vi "Ultramat 23 AFCO Calculations Sub.vi"(7 "CO2 Air Free-Ultimate (%)":dbl, 8 "error in (no error)":errorcluster, 10 "CO2 (%)":dbl, 11 "CO (PPMv)":dbl) -> (0 "error out":errorcluster, 3 "AFCO Data":string[][](array[string]))   [LabVIEW 2023]
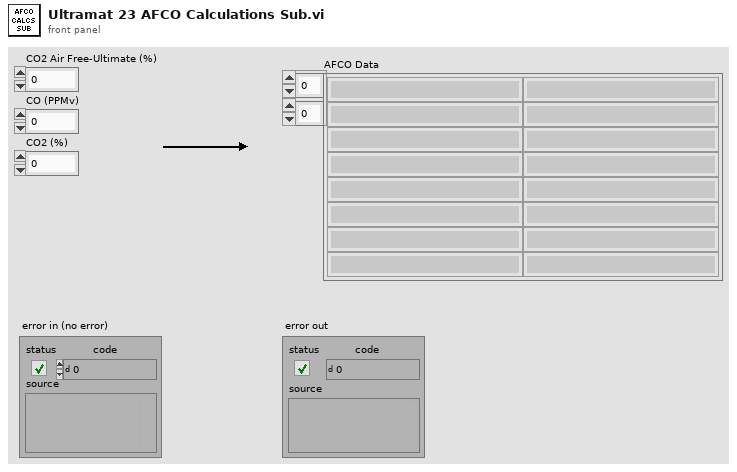
[diagram p1: front panel]
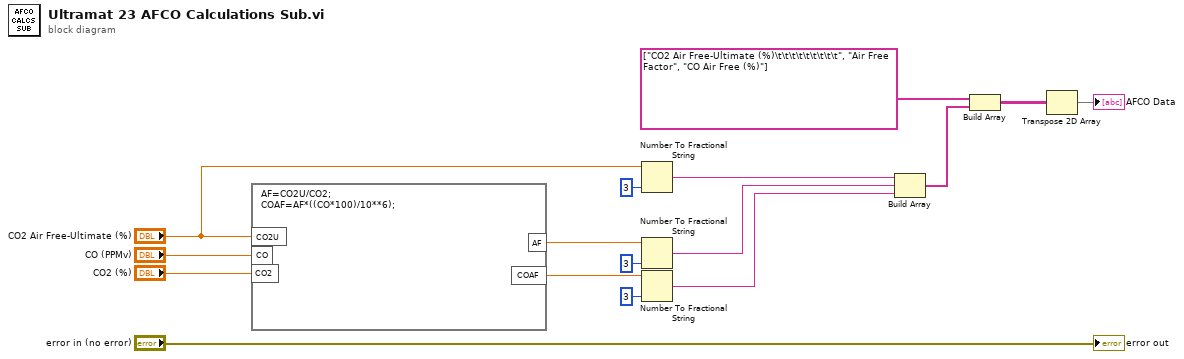
[diagram p0: block diagram]
diagram:
  n1 = formula code="AF=CO2U/CO2;\nCOAF=AF*((CO*100)/10**6);"("CO2U"="CO2 Air Free-Ultimate (%)", "CO"="CO (PPMv)", "CO2"="CO2 (%)") -> ("AF"=w8:dbl, "COAF"=w9:dbl)
  n2 = Number To Fractional String(number="CO2 Air Free-Ultimate (%)", precision (6)=i16 3) -> (F-format string=w10:string)  [unwired: 2 in]
  n3 = Number To Fractional String(number=w8, precision (6)=i16 3) -> (F-format string=w11:string)  [unwired: 2 in]
  n4 = Number To Fractional String(number=w9, precision (6)=i16 3) -> (F-format string=w12:string)  [unwired: 2 in]
  n5 = Build Array(w10, w11, w12) -> (w14:string[])
  n6 = Build Array(string[] ["CO2 Air Free-Ultimate (%)\t\t\t\t\t\t\t\t\t", "Air Free Factor", "CO Air Free (%)"], w14) -> (w15:string[][])
  n7 = Transpose 2D Array(2D array=w15) -> (transposed array=→"AFCO Data":string[][])
  "error out" <- "error in (no error)"
